vi "LimeLightAlignment.vi"() -> (1 "TX":dbl=-21.93614730860138, 3 "Correction":dbl=-0.7)   [LabVIEW 2018]
uses:
  <vilib>/Rock Robotics/Network Tables/NT Write Number.vi
  <vilib>/Rock Robotics/Network Tables/NT Read Number.vi
  <vilib>/addons/control/pid/pid.llb/PID Control Input Filter (DBL).vi
  <vilib>/addons/control/pid/pid.llb/PID (DBL).vi
  LimeLight.vi
  <vilib>/addons/control/pid/NI_PID_pid.lvlib
panel:
  in  "output range":cluster{"output high":dbl, "output low":dbl}={"output high"=0.7, "output low"=-0.7} {"output low" format="%.2f"; "output high" format="%.2f"}
  in  "PID gains":T1={"proportional gain (Kc)"=0.09, "integral time (Ti, min)"=0.03, "derivative time (Td, min)"=0.002} {"proportional gain (Kc)" step=0.01}
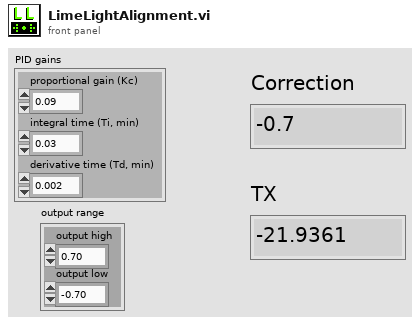
[diagram p1: front panel]
types:
  T1 = cluster{"proportional gain (Kc)":dbl, "integral time (Ti, min)":dbl, "derivative time (Td, min)":dbl}
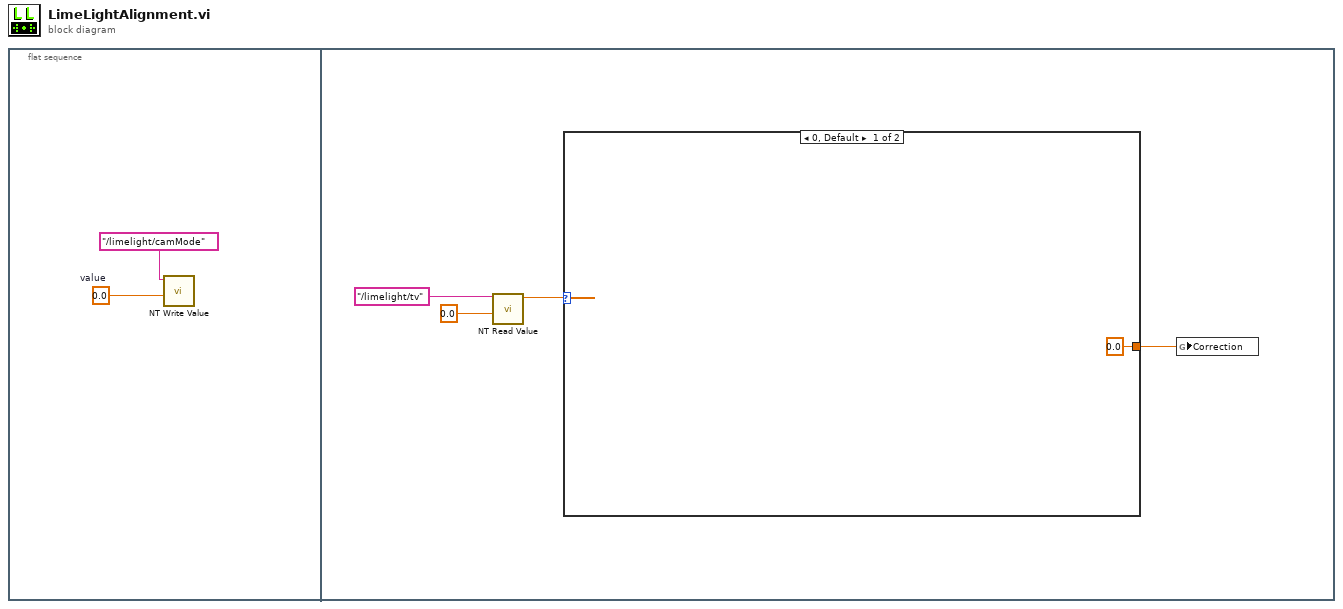
[diagram p0: block diagram]
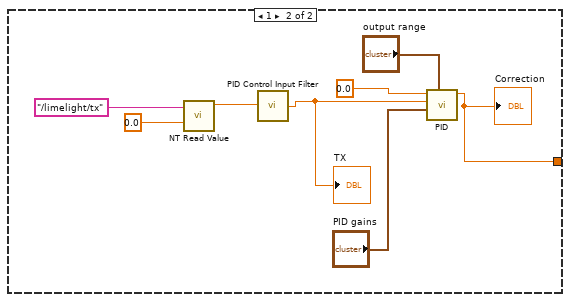
[diagram p2: hidden frame]
diagram:
  n1 = flat-sequence {
    frame #0 {
      w1 = 0.0  # value
      n2 = call-poly <vilib>:"NT Write Value.vi"("Numeric"=w1, "Name"="/limelight/camMode") -> ()  [unwired: 9 in, 1 out]
    }
    frame #1 {
      n3 = call-poly <vilib>:"NT Read Value.vi"("Default Value"=0.0, "Name"="/limelight/tv") -> ("Numeric"=w5:dbl)  [unwired: 8 in, 1 out]
      n4 = case shown="0, Default" w5 {
        tunnel: [0.0 ("output") w9] -> w6
        frame 0, Default {
        }
        frame 1 {
          n5 = call-poly <vilib>:"NT Read Value.vi"("Default Value"=0.0, "Name"="/limelight/tx") -> ("Numeric"=w11:dbl)  [unwired: 8 in, 1 out]
          n6 = call-poly <vilib>:"PID Control Input Filter.vi"("input"=w11) -> ("output"=w10:dbl)  [unwired: 4 in]
          "TX" <- w10
          n7 = call-poly <vilib>:"PID.vi"("output range"="output range", "PID gains"="PID gains", "process variable"=w10, "setpoint"=0.0) -> ("output"=w9:dbl)  [unwired: 6 in, 1 out]
          "Correction" <- w9
        }
      }
      n8 = global write "LimeLight.vi" "Correction"(w6) -> ()
    }
  }
